vi "220426_y7x1_cappture.vi"(4 "start Col.":dbl, 5 "Rawdata pixmap":u8[][](array[numeric])=array40x561[22440 elements] caption="Input pixmap") -> (0 "TapN":dbl, 1 "moving Log(Y, X)":i32[][](array[numeric]), 2 "Total point":i32)   [LabVIEW 2016]
panel:
  out "point log":i32[](array[numeric])
  out "vertical":i32
  # "How to use : \nΔ = (vertical 40) / (23-22) ) = 40 \nΔ = (vertical 20) / (30-20) ) =  2 \nΔ = (vertical 35) / (23-20) ) = 11.67"
  # "Round (i / 11.67)\n  i  : prog. \n  0 : 0\n  1 : 0\n  4 : 0\n  5 : 1\n17 : 1\n18 : 2\n29 : 2\n30 : 3\n35 : 3"
  # "Δ ="
  # "="
  # "ー"
  # "progress = Round( i / Δ ) ="
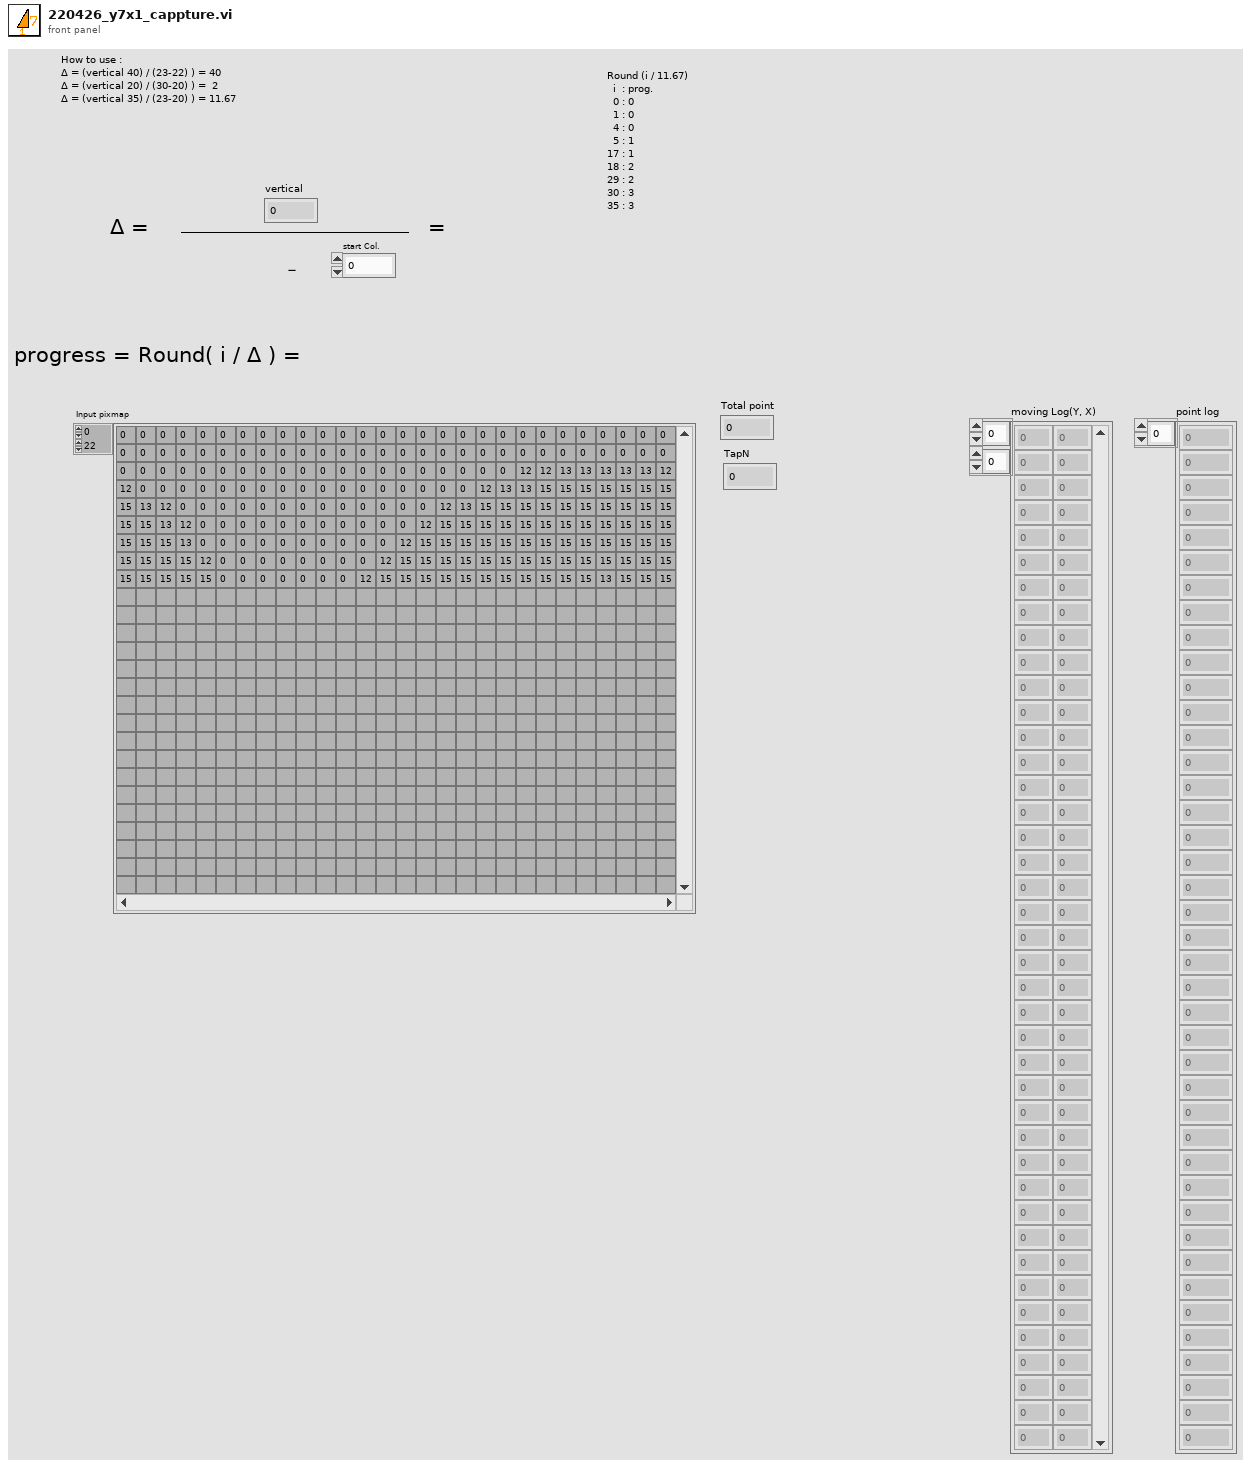
[diagram p1: front panel]
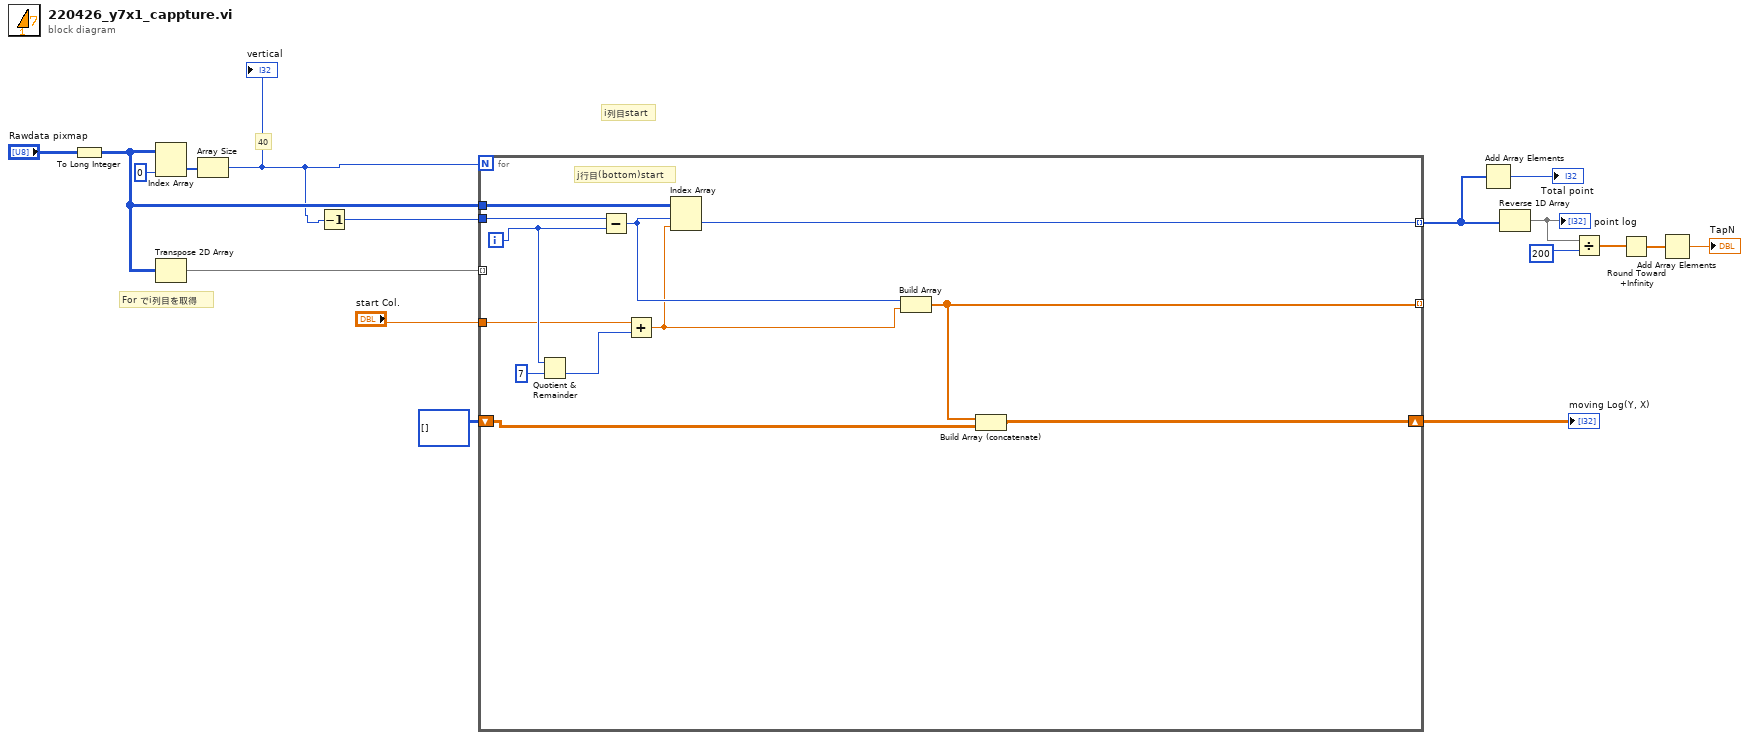
[diagram p0: block diagram]
diagram:
  # "i列目start"
  # "40"
  # "For でi列目を取得"
  n1 = To Long Integer(number="Rawdata pixmap") -> (32bit integer=w14:i32[][])
  n2 = Index Array(array=w14, index (col)=0 ("無効な指標 （列）")) -> (element=w15:i32[])  [unwired: 1 in]
  n3 = Transpose 2D Array(2D array=w14) -> (transposed array=w13:i32[][])
  n4 = Array Size(array=w15) -> (size(s)=w8:i32)
  "vertical" <- w8
  n5 = Decrement(x=w8) -> (x-1=w11:i32)
  n6 = for {
    N: w8 -> [_]
    tunnel: w13 -> [_] mode=indexing
    tunnel: w11 -> [w28]
    tunnel: w14 -> [w29]
    tunnel: [w27] -> w7 mode=indexing
    tunnel: [w23] -> _ mode=indexing
    shift-right: [w24] -> w9
    shift-left: i32[][] [] -> [w22]
    tunnel: "start Col." -> [w18]
    i -> [w21]
    # "j行目(bottom)start"
    n7 = Quotient & Remainder(x=w21, y=7) -> (floor(x/y)=w19:i32)  [unwired: 1 out]
    n8 = Subtract(x=w28, y=w21) -> (x-y=w26:i32)
    n9 = Add(x=w18, y=w19) -> (x+y=w25:dbl)
    n10 = Index Array(array=w29, index (row)=w26, index (col)=w25) -> (element=w27:i32)
    n11 = Build Array(w26, w25) -> (w23:dbl[])
    n12 = Build Array (concatenate)(w23, w22) -> (w24:dbl[][])
  }
  "moving Log(Y, X)" <- w9
  n13 = Add Array Elements(numeric array=w7) -> (sum=→"Total point":i32)
  n14 = Reverse 1D Array(array=w7) -> (reversed array=w6:i32[])
  "point log" <- w6
  n15 = Divide(x=w6, y=200) -> (x/y=w4:dbl[])
  n16 = Round Toward +Infinity(x=w4) -> (ceil(x): smallest int >= x=w3:dbl[])
  n17 = Add Array Elements(numeric array=w3) -> (sum=→"TapN":dbl)
